vi "Map Class.vi"(8 "error in (no error)":errorcluster, 9 "Name":string, 10 "Class object":refnum<class>, 11 "Application Controller in":refnum<class "Application Controller.lvclass">) -> (0 "error out":errorcluster, 3 "Application Controller out":refnum<class "Application Controller.lvclass">)   [LabVIEW 2021, in "Application Controller.lvclass"]
uses:
  Application Controller.lvclass
  Application Controller.lvclass/Application Controller.ctl
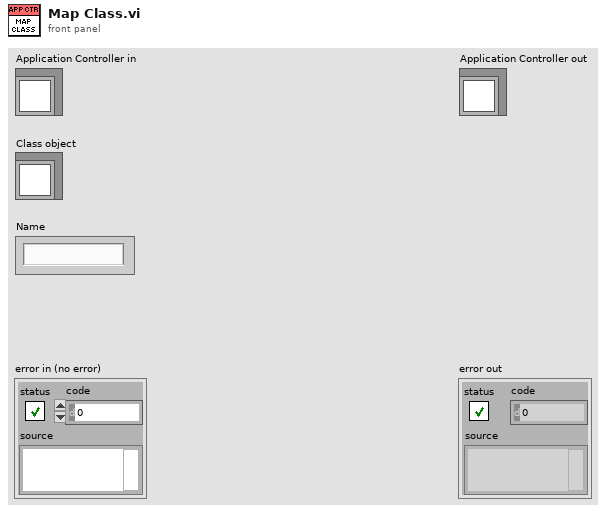
[diagram p1: front panel]
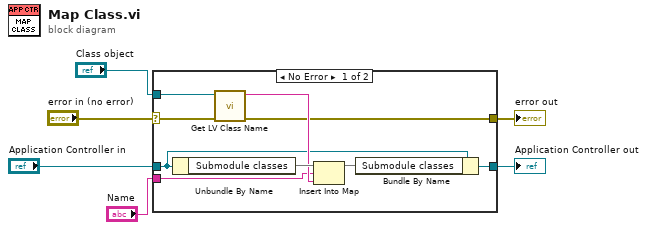
[diagram p0: block diagram]
diagram:
  n1 = case shown="No Error" "error in (no error)" {
    selector: "error in (no error)" -> [w8 w17]
    tunnel: [w7 w17] -> w5
    tunnel: [w10 w16] -> w3
    tunnel: "Application Controller in" -> [w11 w16]
    tunnel: "Name" -> [w12 _]
    tunnel: "Class object" -> [w9 _]
    frame No Error {
      n2 = Unbundle By Name(w11) -> ("Submodule classes"=w14:map{string, string})
      n3 = call <vilib>:"Get LV Class Name.vi"("error in (no error)"=w8, "object"=w9) -> ("error out"=w7:errorcluster, "class name"=w13:string)  [unwired: 8 in]
      n4 = Insert Into Map(map in=w14, key=w12, value=w13) -> (map out=w15:map{string, string})  [unwired: 2 out]
      n5 = Bundle By Name(cluster=w11, "Submodule classes"=w15) -> (w10:refnum<class "Application Controller.lvclass">)
    }
    frame Error {
    }
  }
  "error out" <- w5
  "Application Controller out" <- w3
